vi "ArrayToString_Sushu.vi"(11 "Array":string[](array[string])) -> (3 "String":string)   [LabVIEW 2017, in "sushu.lvlib"]
doc: "字符串数组转换为单个字符串（一行行）。\n2014-09-17 12:57:44\n蒋松\njiangsong@outlook.com"
uses:
  <userlib>/sushu/sushu.lvlib
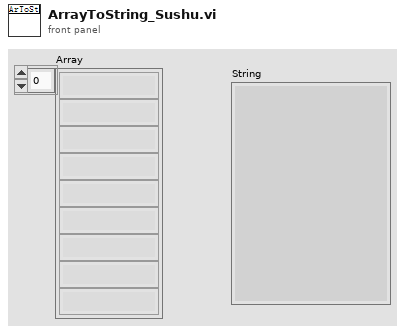
[diagram p1: front panel]
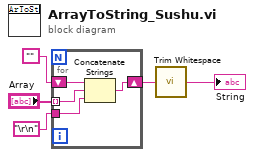
[diagram p0: block diagram]
diagram:
  n1 = for {
    tunnel: "Array" -> [w8] mode=indexing
    shift-right: [w6] -> w2
    shift-left: "" -> [w9]
    tunnel: "\r\n" -> [w7]
    n2 = Concatenate Strings(w9, w8, w7) -> (w6:string)
  }
  n3 = call <vilib>:"Trim Whitespace.vi"("string"=w2) -> ("trimmed string"=→"String":string)  [unwired: 1 in]
